vi "tmdsverify.vi"(11 "file path":path) -> (3 "Boolean":bool)   [LabVIEW 2015]
panel:
  out "Numeric":dbl
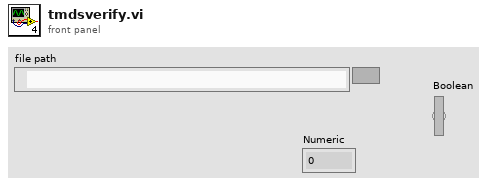
[diagram p1: front panel]
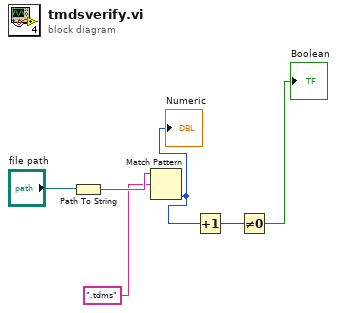
[diagram p0: block diagram]
diagram:
  n1 = Path To String(path="file path") -> (string=w5:string)
  n2 = Match Pattern(string=w5, regular expression=".tdms") -> (offset past match=w2:i32)  [unwired: 1 in, 3 out]
  "Numeric" <- w2
  n3 = Increment(x=w2) -> (x+1=w1:i32)
  n4 = Not Equal To 0?(x=w1) -> (x != 0?=→"Boolean":bool)
